vi "Process.vi"(8 "error in":errorcluster, 11 "HAL":refnum<class "HAL.lvclass">) -> (0 "error out":errorcluster, 3 "HAL out":refnum<class "HAL.lvclass">)   [LabVIEW 2019, in "Instrument.lvlib" / "HAL.lvclass"]
uses:
  HAL.lvclass
  C:/Program Files (x86)/National Instruments/LabVIEW 2019/vi.lib/JKI/JKI SMO/SMO/SMO.lvclass
  <vilib>/JKI/JKI SMO/SMO/SMO.lvclass/SMO.ctl
  <vilib>/JKI/JKI SMO/SMO/Private/ReftoDVR--SMO.vi
  <vilib>/JKI/JKI SMO/SMO/SMO.lvclass
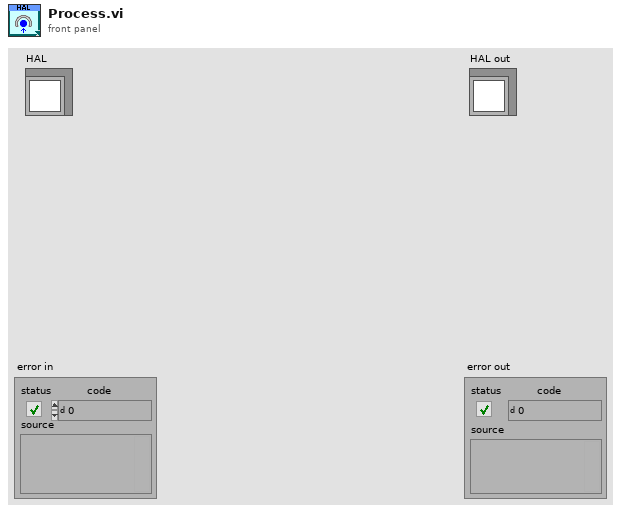
[diagram p1: front panel]
types:
  T1 = enum32{"invalid app kind", "Development System", "Run Time System", "Student Edition", "Embedded LabVIEW", "Evaluation", "Custom"}
  T2 = enum32{"Invalid", "Standard", "Closed", "Hidden", "Minimized", "Maximized"}
  T3 = cluster{"Core":cluster{"Current VI Reference":refnum<vi>, "Close Panel on Exit?":bool, "Last Error":cluster{"error":errorcluster, "previous state":string, "remaining states":string}, "Shutdown?":bool}, "SelfRef":refnum<class "HAL.lvclass">}
  T4 = cluster{"Current VI Reference":refnum<vi>, "Close Panel on Exit?":bool, "Last Error":cluster{"error":errorcluster, "previous state":string, "remaining states":string}, "Shutdown?":bool}
  T5 = typedef "SMO.lvclass/Protected Events.ctl" = cluster{"StopProcesses":refnum<user-event>, "AbortProcesses":refnum<user-event>, "Config Changed":refnum<user-event>, "Dependency":refnum<user-event>}
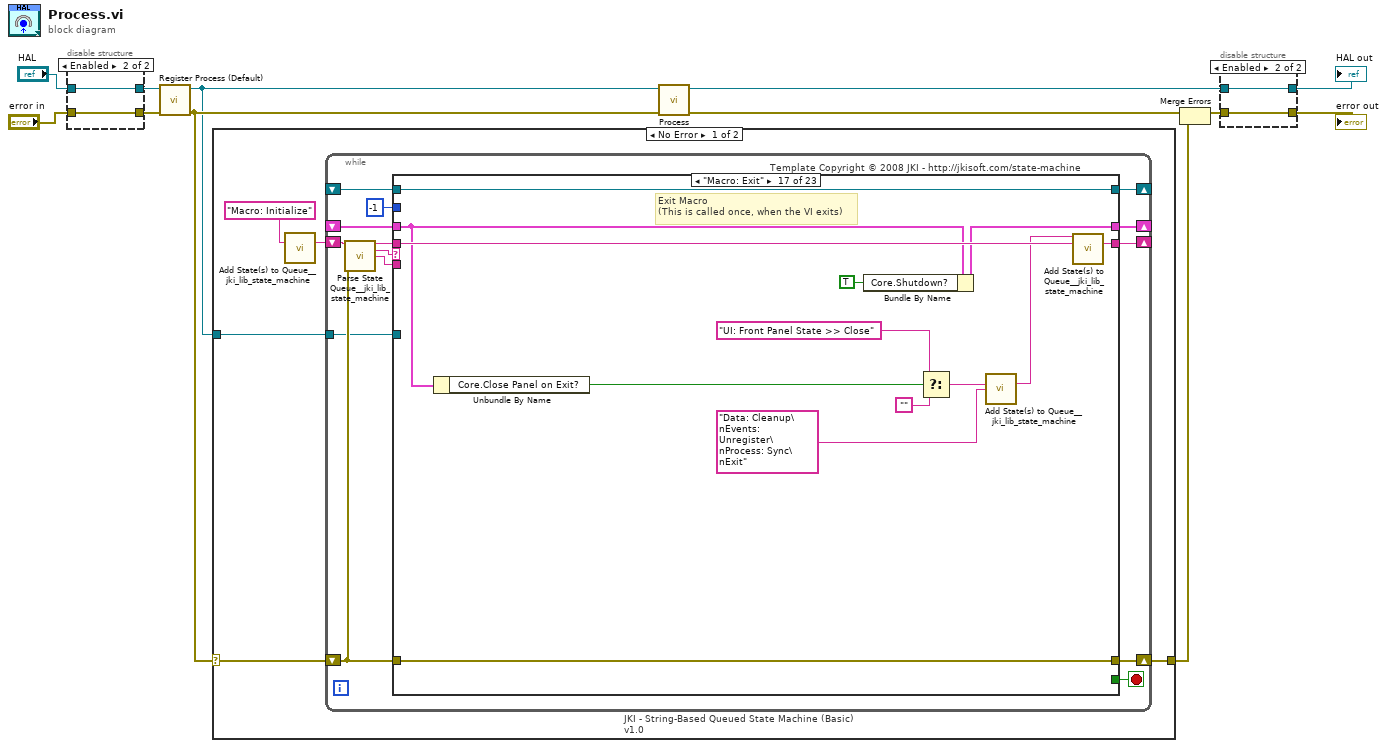
[diagram p0: block diagram]
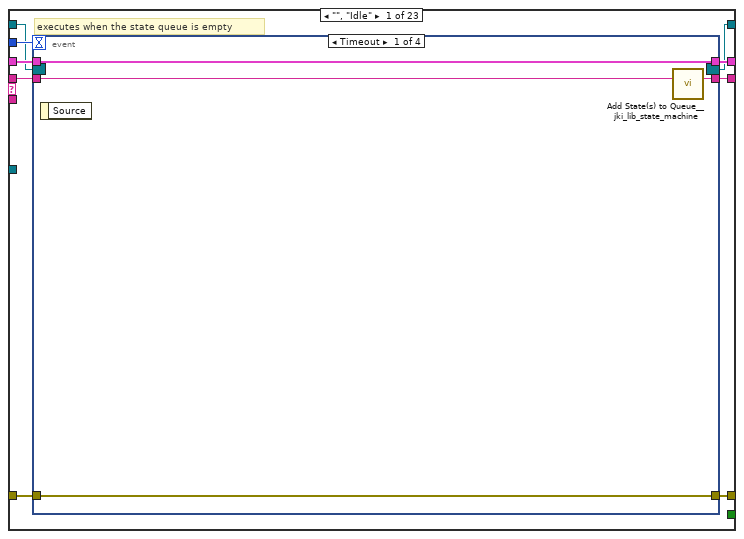
[diagram p4: hidden frame]
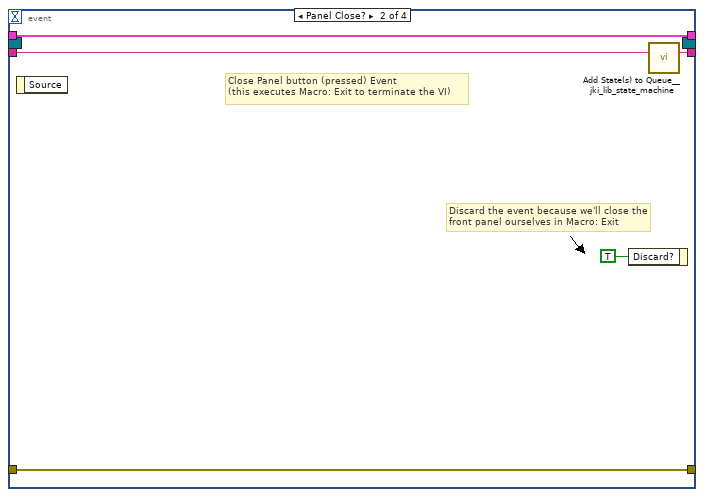
[diagram p5: hidden frame]
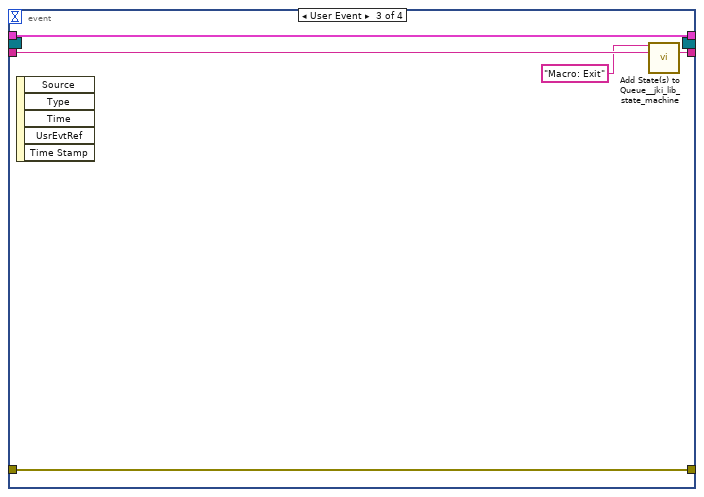
[diagram p6: hidden frame]
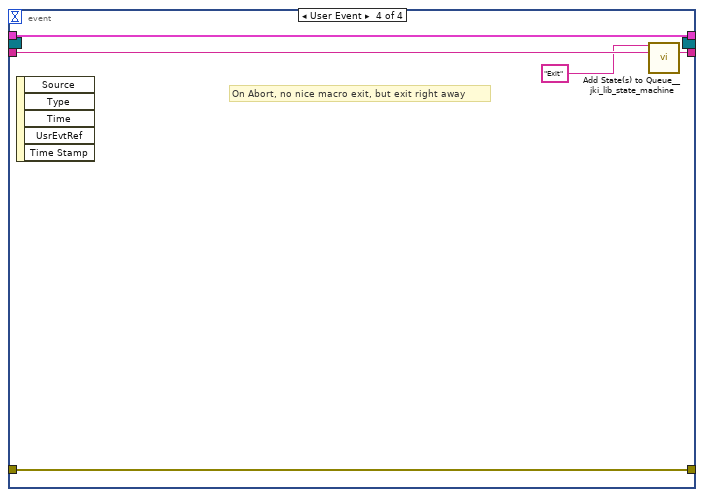
[diagram p7: hidden frame]
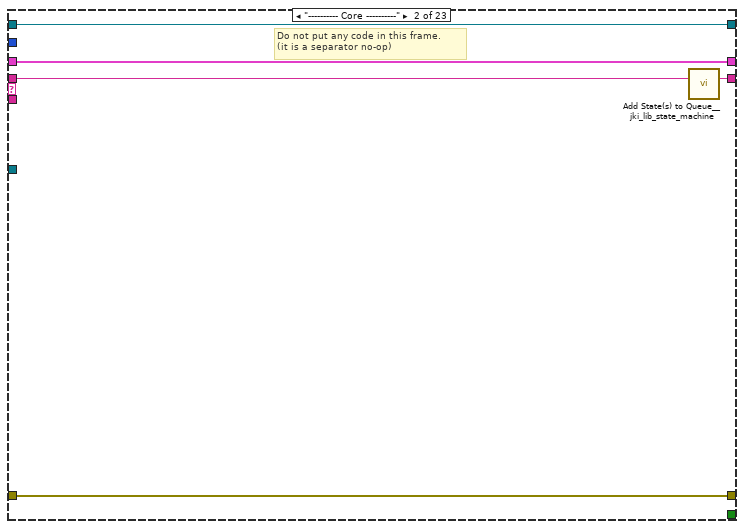
[diagram p8: hidden frame]
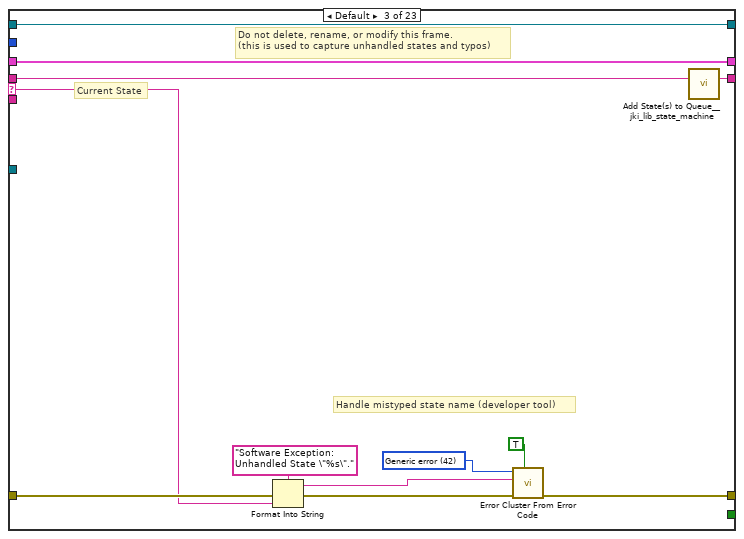
[diagram p9: hidden frame]
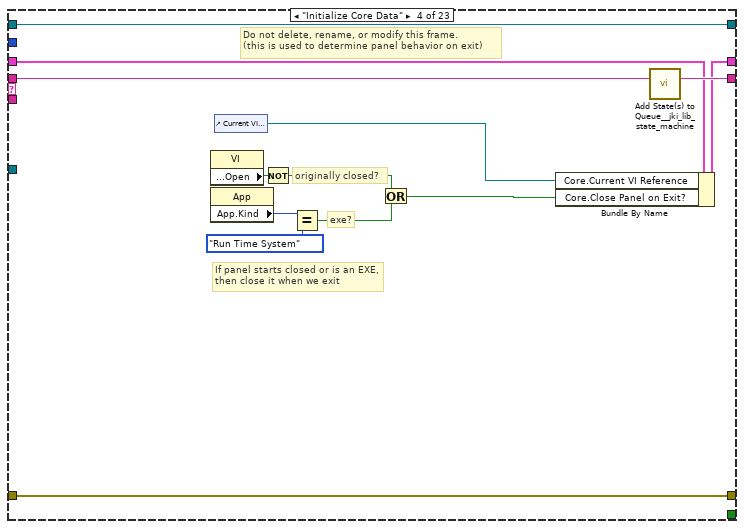
[diagram p10: hidden frame]
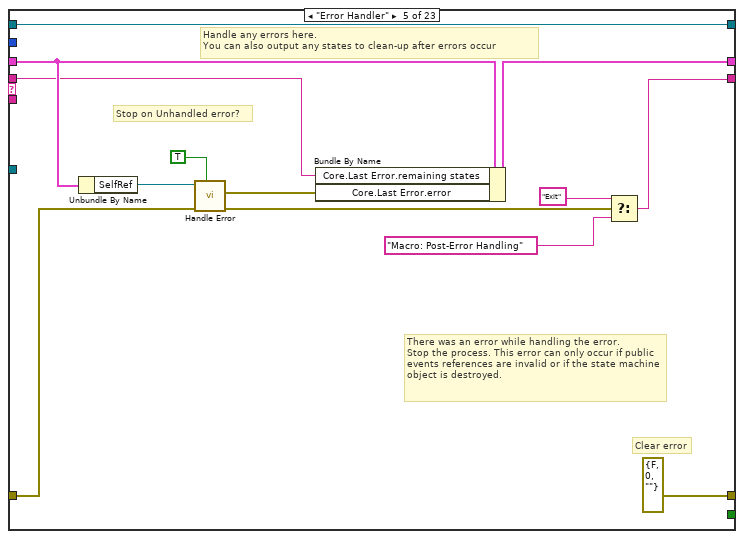
[diagram p11: hidden frame]
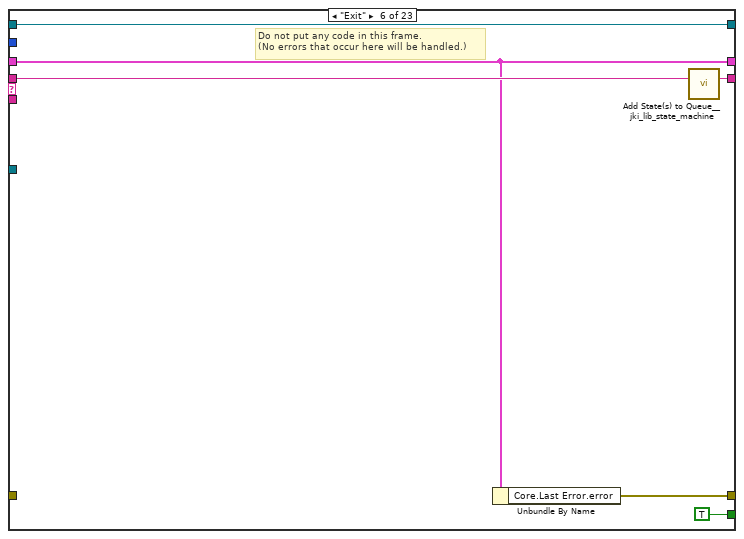
[diagram p12: hidden frame]
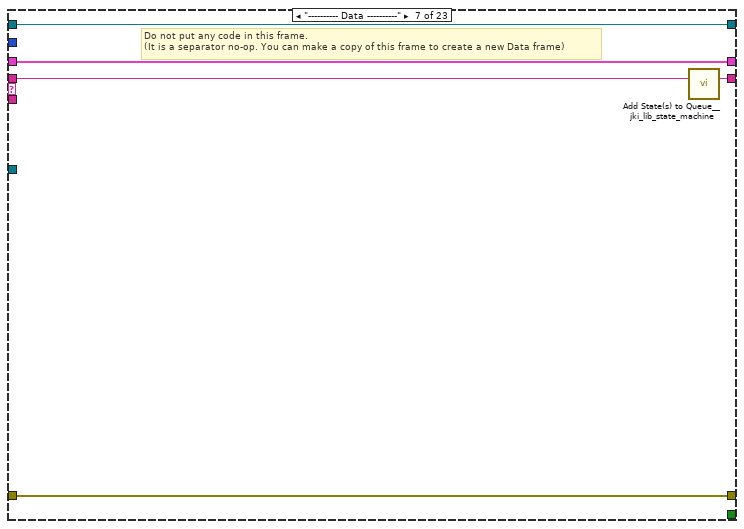
[diagram p13: hidden frame]
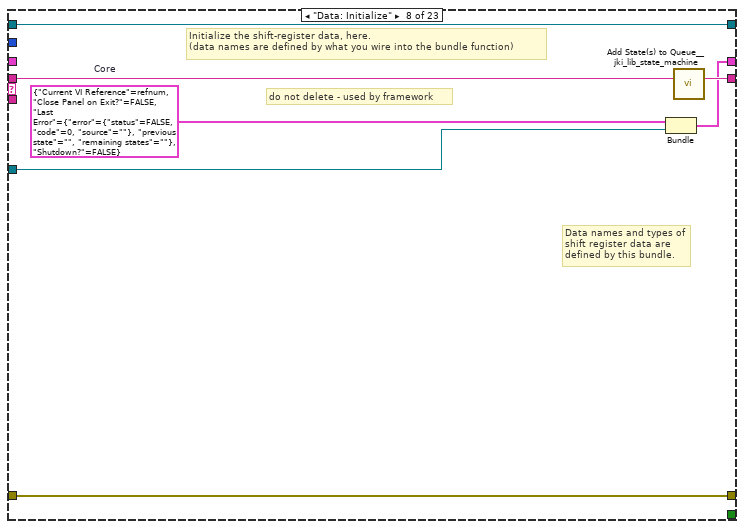
[diagram p14: hidden frame]
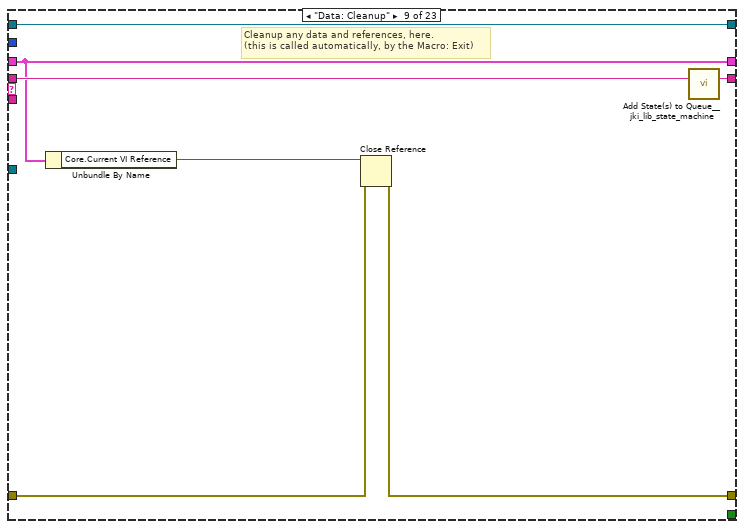
[diagram p15: hidden frame]
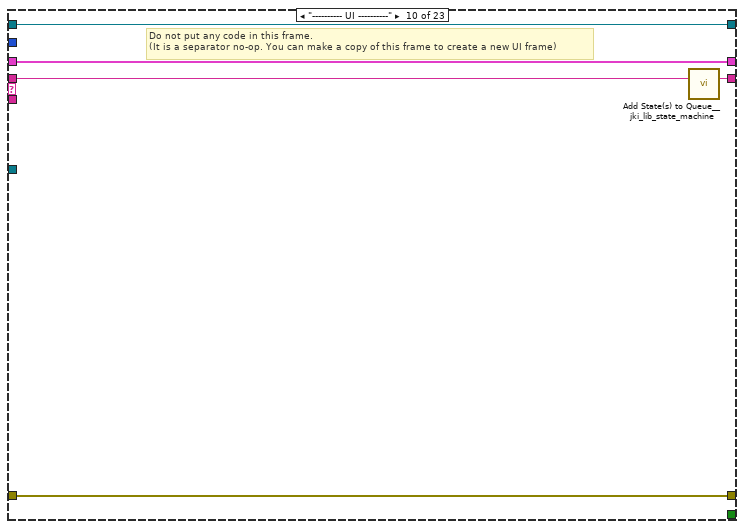
[diagram p16: hidden frame]
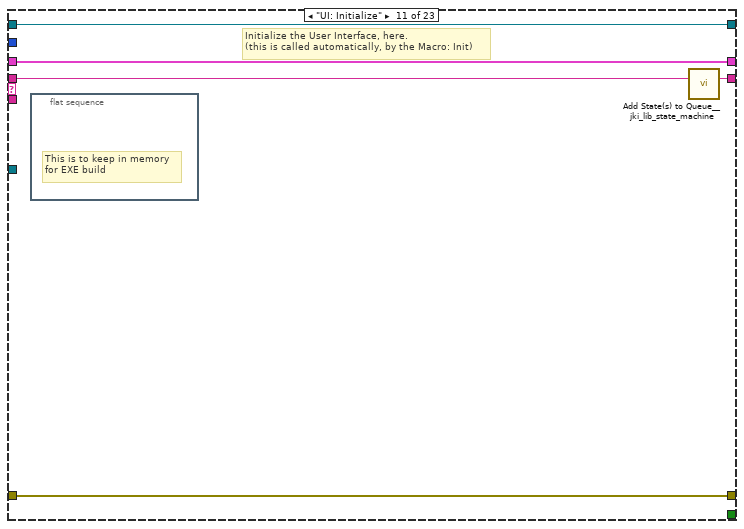
[diagram p17: hidden frame]
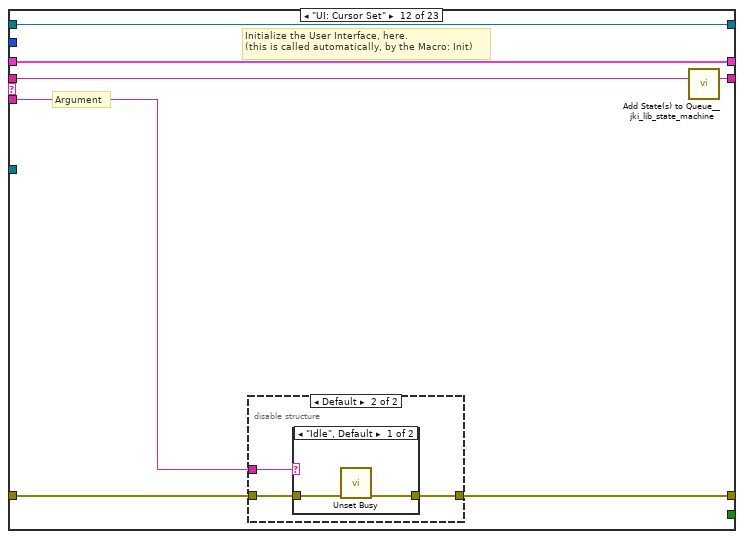
[diagram p18: hidden frame]
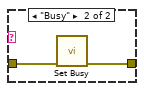
[diagram p20: hidden frame]
diagram:
  n1 = disable-structure shown="Enabled" {
    disable-tunnel: [_ w15] -> w11
    disable-tunnel: [w13 w14] -> w12
    disable-tunnel: "error in" -> [w13 w14]
    disable-tunnel: "HAL" -> [_ w15]
    frame Disabled {
      # "error in"
      # "SMO in"
    }
    frame Enabled {
    }
  }
  n2 = call <vilib>:"Register Process (Default).vi"("error in (no error)"=w12, "SMO"=w11) -> ("error out"=w10:errorcluster, "SelfRef"=w9:refnum<class "HAL.lvclass">)  [unwired: 8 in]
  n3 = case shown="No Error" w10 {
    selector: w10 -> [w19 w276]
    tunnel: w9 -> [w20 _]
    tunnel: [w18 w276] -> w6
    frame No Error {
      n4 = call <vilib>:"Add State(s) to Queue__jki_lib_state_machine.vi"("State(s) in (\"\")"="Macro: Initialize") -> ("States Out"=w16:string)  [unwired: 14 in]
      n5 = while "JKI - String-Based Queued State Machine (Basic) v1.0" {
        shift-right: [w27] -> _
        shift-left: _ -> [w26]
        shift-right: [w30] -> w18
        shift-left: w19 -> [w24]
        shift-right: [w29] -> _
        shift-left: w16 -> [w31]
        tunnel: w20 -> [w23]
        shift-right: [w22] -> _
        shift-left: _ -> [w21]
        stop <- w28 stop-if-true
        # "Template Copyright © 2008 JKI - http://jkisoft.com/state-machine"
        n6 = call <vilib>:"Parse State Queue__jki_lib_state_machine.vi"("State Queue"=w31, "Error In (no error)"=w24) -> ("Remaining States"=w33:string, "Current State"=w34:string, "Arguments"=w32:string)  [unwired: 11 in]
        n7 = case shown="\"Macro: Exit\"" w34 {
          selector: w34 -> [_ _ w69 _ _ _ _ _ _ _ _ _ _ _ _ _ _ _ _ _ _ _ _]
          tunnel: w33 -> [w43 w67 w73 w92 w94 w111 w116 w123 w130 w135 w140 w147 w163 w195 w204 w216 w233 w238 w249 w254 w264 w270 w275]
          tunnel: w32 -> [_ _ _ _ _ _ _ _ _ _ _ w141 w159 _ _ _ _ _ _ _ _ _ _]
          tunnel: w26 -> [w41 w64 w71 w83 w103 w107 w113 _ w125 w132 w138 w145 w161 w192 w200 w208 w223 w235 w246 w251 w262 w268 w272]
          tunnel: [w40 w65 w75 w89 errorcluster {"status"=FALSE, "code"=0, "source"=""} ("error out") w106 w114 w118 w126 w133 w137 w142 w156 w193 w202 w214 w231 w236 w240 w252 w255 w266 w273] -> w30
          tunnel: w24 -> [w39 w65 w74 w89 w100 _ w114 w118 w127 w133 w137 w143 w157 w193 w202 w214 w231 w236 w241 w252 w258 w266 w273]
          tunnel: [w42 w66 w72 w91 w93 w110 w115 w122 w129 w134 w139 w146 w162 w194 w203 w215 w232 w237 w248 w253 w263 w269 w274] -> w29
          tunnel: [_ _ _ _ _ TRUE _ _ _ _ _ _ _ _ _ _ _ _ _ _ _ _ _] -> w28
          tunnel: [w38 w64 w71 w90 w102 w107 w113 w121 w125 w132 w138 w145 w161 w192 w200 w212 w222 w235 w246 w251 w262 w268 w272] -> w27
          tunnel: -1 ("Timeout") -> [w37 _ _ _ _ _ _ _ _ _ _ _ _ _ _ _ _ _ _ _ _ _ _]
          tunnel: w23 -> [_ _ _ _ _ _ _ w117 _ _ _ _ _ _ _ _ _ _ _ _ _ _ _]
          tunnel: [w35 w63 w68 w80 w105 w108 w112 w120 w124 w131 w136 w144 w160 w191 w201 w213 w225 w234 w247 w250 w260 w267 w271] -> w22
          tunnel: w21 -> [w36 w63 w68 w80 w105 w108 w112 w120 w124 w131 w136 w144 w160 w191 w201 w213 w225 w234 w247 w250 _ w267 w271]
          frame "", "Idle" {
            # "executes when the state queue is empty"
            n8 = event shown="[0] Timeout" {
              selector: w36 -> [_ _ _ _]
              dyn-events: [_ _ _ _] -> w35
              timeout: w37 -> [_ _ _ _]
              tunnel: w43 -> [w47 w52 w57 w62]
              tunnel: [w46 w51 w56 w61] -> w42
              tunnel: w41 -> [w44 w48 w54 w59]
              tunnel: [w45 w50 w55 w60] -> w40
              tunnel: w39 -> [w45 w50 w55 w60]
              tunnel: [w44 w48 w54 w59] -> w38
              event Timeout {
                n9 = event-data() -> ()  [unwired: 1 in, 1 out]
                n10 = call <vilib>:"Add State(s) to Queue__jki_lib_state_machine.vi"("State(s) in (\"\")"=w47) -> ("States Out"=w46:string)  [unwired: 14 in]
              }
              event Panel Close? {
                # "Discard the event because we'll close the front panel ourselves in Macro: Exit"
                # "Close Panel button (pressed) Event\n(this executes Macro: Exit to terminate the VI)"
                n11 = event-data() -> ()  [unwired: 1 in, 1 out]
                n12 = event-data("Discard?"=TRUE) -> ()  [unwired: 1 in, 1 out]
                n13 = call <vilib>:"Add State(s) to Queue__jki_lib_state_machine.vi"("State(s) in (\"\")"=w52) -> ("States Out"=w51:string)  [unwired: 14 in]
              }
              event User Event {
                n14 = event-data() -> ()  [unwired: 1 in, 5 out]
                n15 = call <vilib>:"Add State(s) to Queue__jki_lib_state_machine.vi"("State(s) in Front (\"\")"="Macro: Exit", "State(s) in (\"\")"=w57) -> ("States Out"=w56:string)  [unwired: 13 in]
              }
              event User Event {
                # "On Abort, no nice macro exit, but exit right away"
                n16 = event-data() -> ()  [unwired: 1 in, 5 out]
                n17 = call <vilib>:"Add State(s) to Queue__jki_lib_state_machine.vi"("State(s) in Front (\"\")"="Exit", "State(s) in (\"\")"=w62) -> ("States Out"=w61:string)  [unwired: 13 in]
              }
            }
          }
          frame "---------- Core ----------" {
            # "Do not put any code in this frame.\n(it is a separator no-op)"
            n18 = call <vilib>:"Add State(s) to Queue__jki_lib_state_machine.vi"("State(s) in (\"\")"=w67) -> ("States Out"=w66:string)  [unwired: 14 in]
          }
          frame Default {
            w78 = 42 items=["No error", "Argument error", "Memory is full", "Out of zone", "End of file", "File already open", "Generic file I/O error", "File not found", "File permission error", "Disk is full", "Duplicate path", "Too many files open", "System feature not enabled", "Resource file not found", "Cannot add resource", "Resource not found", "Image not found", "Image memory error", "Pen does not exist", "Config type invalid", "Config token not found", "Config parse error", "Config memory error", "Bad external code format", "Bad external code offset", "External code not present", "Null window", "Destroy window error", "Null menu", "Print aborted", "Bad print record", "Print driver error", "Windows error during printing", "Memory error during printing", "Print dialog error", "Generic print error", "Invalid device refnum", "Device not found", "Device parameter error", "Device unit error", "Cannot open device", "Device call aborted", "Generic error", "Cancelled by user", "Object ID too low", "Object ID too high", "Object not in heap", "Unknown heap", "Unknown object (invalid DefProc)", "Unknown object (DefProc not in table)", "Message out of range", "Invalid (null) method", "Unknown message", "Manager call not supported", "Bad address", "Network operation in progress", "Network operation timed out", "Connection is busy", "Network attribute not supported", "Network error", "Address in use", "System out of memory", "Connection aborted", "Connection refused", "Not connected", "Already connected", "Connection closed", "Initialization error (interapplication manager)", "Bad occurrence", "Wait on unbound occurrence handler", "Occurrence queue overflow", "Datalog type conflict", "Unused", "Unrecognized type (interapplication manager)", "Memory corrupt", "Failed to make temporary DLL", "Old CIN version", "Drag socket not found", "Failed to load drop-object", "Failed to register OLE object", "Failed to release OLE object", "Format specifier type mismatch", "Unknown format specifier", "Too few format specifiers", "Too many format specifiers", "Scan failed", "Newer CIN version", "Error converting to variant", "Runtime menu error", "Password tampered", "Variant attribute not found", "Incompatible variant data type", "Event data is not available", "Event Store is not present", "Occurrence is not found", "Event Queue is not created", "Event info is not available", "Refnum passed is NULL", "Error retrieving Class GUID", "Error retrieving CoClass GUID", "Error retrieving TypeLib GUID.", "Bad built application magic bytes.", "Specific driver is different from the specific driver associated with the Logical Name.", "There is no session opened to the class driver.", "Max Error", "MAX - Error with config objects", "MAX - Error loading configuration", "MAX - Group not supported"]
            # "Current State"
            # "Do not delete, rename, or modify this frame.\n(this is used to capture unhandled states and typos)"
            # "Handle mistyped state name (developer tool)"
            n19 = Format Into String(format string="Software Exception: Unhandled State \"%s\"." ("message"), error in=w74, w69) -> (resulting string=w77:string, error out=w76:errorcluster)  [unwired: 1 in]
            n20 = call <vilib>:"Error Cluster From Error Code.vi"("show call chain? (False)"=TRUE, "error in (no error)"=w76, "error message (\"\")"=w77, "error code (0)"=w78) -> ("error out"=w75:errorcluster)  [unwired: 5 in]
            n21 = call <vilib>:"Add State(s) to Queue__jki_lib_state_machine.vi"("State(s) in (\"\")"=w73) -> ("States Out"=w72:string)  [unwired: 14 in]
          }
          frame "Initialize Core Data" {
            # "Do not delete, rename, or modify this frame.\n(this is used to determine panel behavior on exit)"
            # "originally closed?"
            # "exe?"
            # "If panel starts closed or is an EXE, then close it when we exit"
            n22 = property class="VI"() -> ("Front Panel.Open"=w88:bool)  [unwired: 2 in, 2 out]
            n23 = property class="App"() -> ("App.Kind"=w87:T1)  [unwired: 2 in, 2 out]
            n24 = control-ref of="Current VI Reference"() -> (w81:refnum<vi>)
            n25 = Not(x=w88) -> (.not. x?=w85:bool)
            n26 = Equal?(x=w87, y=T1."Run Time System" ("Application:Kind")) -> (x = y?=w84:bool)
            n27 = Or(x=w85, y=w84) -> (x .or. y?=w82:bool)
            n28 = Bundle By Name(cluster=w83, "Core.Current VI Reference"=w81, "Core.Close Panel on Exit?"=w82) -> (w90:T3)
            n29 = call <vilib>:"Add State(s) to Queue__jki_lib_state_machine.vi"("State(s) in (\"\")"=w92) -> ("States Out"=w91:string)  [unwired: 14 in]
          }
          frame "Error Handler" {
            # "Stop on Unhandled error?"
            # "There was an error while handling the error.\nStop the process. This error can only occur if public events references are invalid or if the state machine object is destroyed."
            # "Handle any errors here.\nYou can also output any states to clean-up after errors occur"
            # "Clear error"
            n30 = Unbundle By Name(w103) -> ("SelfRef"=w104:refnum<class "HAL.lvclass">)
            n31 = call-dynamic "Handle Error.vi"("Stop on Unhandled Error (T)"=TRUE, "error in"=w100, "SMO"=w104) -> ("handling error"=w98:errorcluster, "Unhandled error"=w101:errorcluster)  [unwired: 6 in, 1 out]
            n32 = Bundle By Name(cluster=w103, "Core.Last Error.remaining states"=w94, "Core.Last Error.error"=w101) -> (w102:T3)
            n33 = Select(t="Exit", s=w98, f="Macro: Post-Error Handling") -> (s? t:f=w93:string)
          }
          frame "Exit" {
            # "Do not put any code in this frame.\n(No errors that occur here will be handled.)"
            n34 = Unbundle By Name(w107) -> ("Core.Last Error.error"=w106:errorcluster)
            n35 = call <vilib>:"Add State(s) to Queue__jki_lib_state_machine.vi"("State(s) in (\"\")"=w111) -> ("States Out"=w110:string)  [unwired: 14 in]
          }
          frame "---------- Data ----------" {
            # "Do not put any code in this frame.\n(It is a separator no-op. You can make a copy of this frame to create a new Data frame)"
            n36 = call <vilib>:"Add State(s) to Queue__jki_lib_state_machine.vi"("State(s) in (\"\")"=w116) -> ("States Out"=w115:string)  [unwired: 14 in]
          }
          frame "Data: Initialize" {
            w119 = T4 {"Current VI Reference"=refnum, "Close Panel on Exit?"=FALSE, "Last Error"={"error"={"status"=FALSE, "code"=0, "source"=""}, "previous state"="", "remaining states"=""}, "Shutdown?"=FALSE}  # Core
            # "do not delete - used by framework"
            # "Data names and types of shift register data are defined by this bundle."
            # "Initialize the shift-register data, here.\n(data names are defined by what you wire into the bundle function)"
            n37 = Bundle("Core"=w119, "SelfRef"=w117) -> (w121:T3)  [unwired: 1 in]
            n38 = call <vilib>:"Add State(s) to Queue__jki_lib_state_machine.vi"("State(s) in (\"\")"=w123) -> ("States Out"=w122:string)  [unwired: 14 in]
          }
          frame "Data: Cleanup" {
            # "Cleanup any data and references, here.\n(this is called automatically, by the Macro: Exit)"
            n39 = Unbundle By Name(w125) -> ("Core.Current VI Reference"=w128:refnum<vi>)
            n40 = Close Reference(reference=w128, error in (no error)=w127) -> (error out=w126:errorcluster)
            n41 = call <vilib>:"Add State(s) to Queue__jki_lib_state_machine.vi"("State(s) in (\"\")"=w130) -> ("States Out"=w129:string)  [unwired: 14 in]
          }
          frame "---------- UI ----------" {
            # "Do not put any code in this frame.\n(It is a separator no-op. You can make a copy of this frame to create a new UI frame)"
            n42 = call <vilib>:"Add State(s) to Queue__jki_lib_state_machine.vi"("State(s) in (\"\")"=w135) -> ("States Out"=w134:string)  [unwired: 14 in]
          }
          frame "UI: Initialize" {
            # "Initialize the User Interface, here.\n(this is called automatically, by the Macro: Init)"
            n43 = flat-sequence {
              frame #0 {
                # "This is to keep in memory\nfor EXE build"
              }
            }
            n44 = call <vilib>:"Add State(s) to Queue__jki_lib_state_machine.vi"("State(s) in (\"\")"=w140) -> ("States Out"=w139:string)  [unwired: 14 in]
          }
          frame "UI: Cursor Set" {
            # "Argument"
            # "Initialize the User Interface, here.\n(this is called automatically, by the Macro: Init)"
            n45 = disable-structure shown="Default" {
              disable-tunnel: w143 -> [w148 w151]
              disable-tunnel: [w148 w150] -> w142
              disable-tunnel: w141 -> [_ w149]
              frame condition #0 {
              }
              frame condition #1 (active) {
                n46 = case shown="\"Idle\", Default" w149 {
                  tunnel: w151 -> [w153 w155]
                  tunnel: [w152 w154] -> w150
                  frame "Idle", Default {
                    n47 = call <vilib>:"Unset Busy.vi"("error in (no error)"=w153) -> ("error out"=w152:errorcluster)  [unwired: 10 in]
                  }
                  frame "Busy" {
                    n48 = call <vilib>:"Set Busy.vi"("error in (no error)"=w155) -> ("error out"=w154:errorcluster)  [unwired: 9 in, 1 out]
                  }
                }
              }
            }
            n49 = call <vilib>:"Add State(s) to Queue__jki_lib_state_machine.vi"("State(s) in (\"\")"=w147) -> ("States Out"=w146:string)  [unwired: 14 in]
          }
          frame "UI: Front Panel State" {
            # "Argument"
            # "Set Front Panel Open or Closed\n(Usage: \"UI: Front Panel State >> Open|Close\")"
            n50 = Unbundle By Name(w161) -> ("Core.Current VI Reference"=w158:refnum<vi>)
            n51 = disable-structure shown="Default" {
              disable-tunnel: w157 -> [w167 w190]
              disable-tunnel: [w166 w190] -> w156
              disable-tunnel: w158 -> [w165 _]
              disable-tunnel: w159 -> [w164 _]
              frame condition #0 (active) {
                n52 = case shown="\"Open\"" w164 {
                  tunnel: w167 -> [w171 w184]
                  tunnel: [w173 w185] -> w166
                  tunnel: w165 -> [w172 w182]
                  frame "Open" {
                    # "Open FP if not open or invalid"
                    n53 = property class="VI"(reference=w172, error in=w171) -> (reference out=w169:refnum<vi>, error out=w170:errorcluster, "FP.State"=w168:T2)
                    n54 = case shown="Default" w168 {
                      tunnel: [w176 w179] -> w173
                      tunnel: w170 -> [w175 w179]
                      tunnel: w169 -> [w174 _]
                      frame Default {
                        n55 = invoke class="VI" method="FP.Open"(reference=w174, error in=w175, "Activate"=TRUE, "State"=T2."Standard") -> (error out=w176:errorcluster)  [unwired: 1 in, 4 out]
                      }
                      frame "Invalid", "Standard" {
                      }
                    }
                  }
                  frame "Close", Default {
                    # "Close FP is not Closed or Invalid"
                    n56 = property class="VI"(reference=w182, error in=w184) -> (reference out=w181:refnum<vi>, error out=w183:errorcluster, "FP.State"=w180:T2)
                    n57 = case shown="Default" w180 {
                      tunnel: [w186 w189] -> w185
                      tunnel: w183 -> [w186 w188]
                      tunnel: w181 -> [_ w187]
                      frame "Invalid", "Closed" {
                      }
                      frame Default {
                        n58 = invoke class="VI" method="FP.Close"(reference=w187, error in=w188) -> (error out=w189:errorcluster)  [unwired: 1 in, 2 out]
                      }
                    }
                  }
                }
              }
              frame condition #1 {
              }
            }
            n59 = call <vilib>:"Add State(s) to Queue__jki_lib_state_machine.vi"("State(s) in (\"\")"=w163) -> ("States Out"=w162:string)  [unwired: 14 in]
          }
          frame "---------- Macro ----------" {
            # "Do not put any code in this frame.\n(It is a separator no-op. You can make a copy of this frame to create a new Macro frame)"
            n60 = call <vilib>:"Add State(s) to Queue__jki_lib_state_machine.vi"("State(s) in (\"\")"=w195) -> ("States Out"=w194:string)  [unwired: 14 in]
          }
          frame "Macro: Initialize" {
            w198 = "UI: Initialize\nUI: Front Panel State >> Close"  # UI: Initialize UI: Front Panel State >> Close
            # "Initialization Macro\n(This is called once, when the VI starts)"
            n61 = call <vilib>:"Add State(s) to Queue__jki_lib_state_machine.vi"("State(s) in Front (\"\")"="Data: Initialize\nInitialize Core Data\nEvents: Register", "State(s) in (\"\")"="Process: Sync", "State(s) at Back (\"\")"=w198) -> ("States Out"=w197:string)  [unwired: 12 in]
            n62 = call <vilib>:"Add State(s) to Queue__jki_lib_state_machine.vi"("State(s) in Front (\"\")"=w197, "State(s) in (\"\")"=w204) -> ("States Out"=w203:string)  [unwired: 13 in]
          }
          frame "Macro: Post-Error Handling" {
            # "Clear Last Error?"
            n63 = Unbundle By Name(w208) -> ("Core.Last Error.remaining states"=w206:string, "Core.Shutdown?"=w207:bool)
            n64 = Unbundle By Name(w208) -> ("Core.Last Error.error"=w211:errorcluster)
            n65 = case shown="False" FALSE {
              tunnel: w211 -> [w220 _]
              tunnel: [w220 _] -> w210
              frame False {
              }
              frame True {
              }
            }
            n66 = case shown="True" w207 {
              tunnel: w206 -> [w217 w219]
              tunnel: [w217 w218] -> w205
              frame False {
                # "These are the remaining states (at the moment the error occured). States can be altered according to business logic."
                # "NOT SHUTTING DOWN"
              }
              frame True {
                # "Developer can decide to alter the states but should be aware that during the shutdown process, there are certain states that must be run for the SMO to properly shut itself (and this process) down. As such, one can add states to perform additional clean-ups, but should append the remaining state to be executed."
                # "SHUTTING DOWN"
                n67 = call <vilib>:"Add State(s) to Queue__jki_lib_state_machine.vi"("State(s) in (\"\")"=w219) -> ("States Out"=w218:string)  [unwired: 14 in]
              }
            }
            n68 = Bundle By Name(cluster=w208, "Core.Last Error.error"=w210) -> (w212:T3)
            n69 = call <vilib>:"Add State(s) to Queue__jki_lib_state_machine.vi"("State(s) in Front (\"\")"=w205, "State(s) in (\"\")"=w216) -> ("States Out"=w215:string)  [unwired: 13 in]
          }
          frame "Macro: Exit" {
            # "Exit Macro\n(This is called once, when the VI exits)"
            n70 = Unbundle By Name(w223) -> ("Core.Close Panel on Exit?"=w230:bool)
            n71 = Bundle By Name(cluster=w223, "Core.Shutdown?"=TRUE) -> (w222:T3)
            n72 = Select(t="UI: Front Panel State >> Close", s=w230, f="") -> (s? t:f=w227:string)
            n73 = call <vilib>:"Add State(s) to Queue__jki_lib_state_machine.vi"("State(s) in (\"\")"=w227, "State(s) at Back (\"\")"="Data: Cleanup\nEvents: Unregister\nProcess: Sync\nExit") -> ("States Out"=w226:string)  [unwired: 13 in]
            n74 = call <vilib>:"Add State(s) to Queue__jki_lib_state_machine.vi"("State(s) in Front (\"\")"=w226, "State(s) in (\"\")"=w233) -> ("States Out"=w232:string)  [unwired: 13 in]
          }
          frame "---------- Process ----------" {
            # "Template Separator\n(You can make a copy of, or modify, this frame)"
            n75 = call <vilib>:"Add State(s) to Queue__jki_lib_state_machine.vi"("State(s) in (\"\")"=w238) -> ("States Out"=w237:string)  [unwired: 14 in]
          }
          frame "Process: Sync" {
            n76 = Unbundle By Name(w246) -> ("SelfRef"=w242:refnum<class "HAL.lvclass">)
            n77 = call <vilib>:"WaitOnProcessSync.vi"("error in (no error)"=w241, "SMO"=w242) -> ("error out"=w240:errorcluster, "Don't run?"=w245:bool)  [unwired: 7 in, 1 out]
            n78 = Select(t="Data: Cleanup\nEvents: Unregister\nExit", s=w245, f="") -> (s? t:f=w239:string)
            n79 = call <vilib>:"Add State(s) to Queue__jki_lib_state_machine.vi"("State(s) in Front (\"\")"=w239, "State(s) in (\"\")"=w249) -> ("States Out"=w248:string)  [unwired: 13 in]
          }
          frame "---------- Events ----------" {
            # "Template Separator\n(You can make a copy of, or modify, this frame)"
            n80 = call <vilib>:"Add State(s) to Queue__jki_lib_state_machine.vi"("State(s) in (\"\")"=w254) -> ("States Out"=w253:string)  [unwired: 14 in]
          }
          frame "Events: Register" {
            n81 = Unbundle By Name(w262) -> ("SelfRef"=w259:refnum<class "HAL.lvclass">)
            n82 = call <vilib>:"GetProtectedEvents.vi"("error in (no error)"=w258, "SMO"=w259) -> ("error out"=w257:errorcluster, "SMO Protected Events"=w261:T5)  [unwired: 7 in, 1 out]
            n83 = register-events(w261) -> (reference out=w260:refnum<event-registration>, error out=w256:errorcluster)  [unwired: 2 in]
            n84 = call <vilib>:"Add State(s) to Queue__jki_lib_state_machine.vi"("State(s) in (\"\")"=w264) -> ("States Out"=w263:string)  [unwired: 14 in]
            n85 = Merge Errors(w257, w256) -> (w255:errorcluster)
          }
          frame "Events: Unregister" {
            n86 = Unregister For Events(event registration refnum=w267, error in=w266) -> (error out=w265:errorcluster)
            n87 = call <vilib>:"Clear Errors.vi"("error in (no error)"=w265) -> ()  [unwired: 5 in, 2 out]
            n88 = call <vilib>:"Add State(s) to Queue__jki_lib_state_machine.vi"("State(s) in (\"\")"=w270) -> ("States Out"=w269:string)  [unwired: 14 in]
          }
          frame "--------- Section ---------" {
            # "Section Separator\n(You can make a copy of, or modify, this frame)"
            n89 = call <vilib>:"Add State(s) to Queue__jki_lib_state_machine.vi"("State(s) in (\"\")"=w275) -> ("States Out"=w274:string)  [unwired: 14 in]
          }
        }
      }
    }
    frame Error {
    }
  }
  n90 = call-parent "Process.vi"("error in"=w10, "SMO"=w9) -> ("error out"=w5:errorcluster, "SMO out"=w8:refnum<class "HAL.lvclass">)  [unwired: 8 in]
  n91 = Merge Errors(w5, w6) -> (w7:errorcluster)
  n92 = disable-structure shown="Enabled" {
    disable-tunnel: w7 -> [_ w277]
    disable-tunnel: w8 -> [_ w278]
    disable-tunnel: [_ w278] -> w2
    disable-tunnel: [_ w277] -> w1
    frame Disabled {
      # "error out"
      # "SMO out"
    }
    frame Enabled {
    }
  }
  "error out" <- w1
  "HAL out" <- w2
